vi "inputToGetList.vi"(8 "error in (no error)":errorcluster, 9 "NumOfDevices":i32, 10 "DeviceConnected":bool, 11 "SEDSpectrometer in":refnum<class "SEDSpectrometer.lvclass">) -> (0 "error out":errorcluster, 1 "ListInput":u8[](array[numeric]), 2 "ListSizeInput":i32, 3 "SEDSpectrometer out":refnum<class "SEDSpectrometer.lvclass">)   [LabVIEW 2016, in "SEDSpectrometer.lvclass"]
uses:
  SEDSpectrometer.lvclass
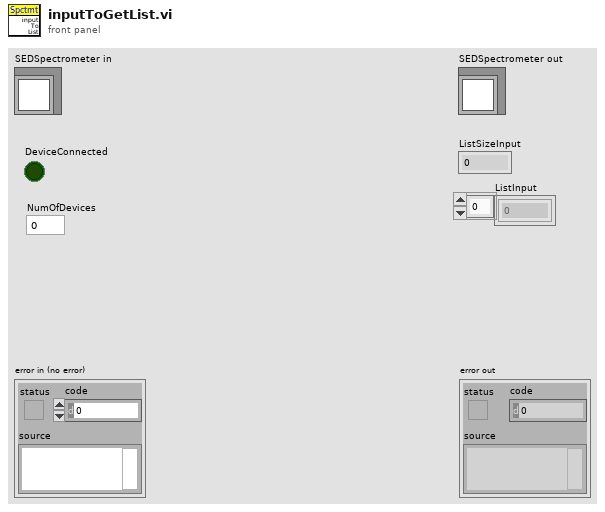
[diagram p1: front panel]
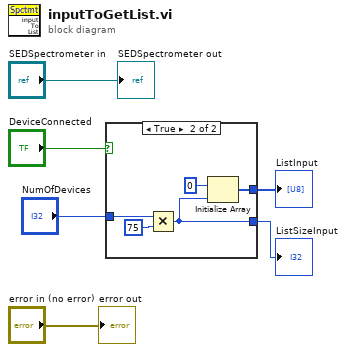
[diagram p0: block diagram]
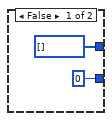
[diagram p2: hidden frame]
diagram:
  n1 = case shown="True" "DeviceConnected" {
    tunnel: "NumOfDevices" -> [_ w13]
    tunnel: [u8[] [] w10] -> w2
    tunnel: [0 w9] -> w1
    frame False {
    }
    frame True {
      n2 = Multiply(x=w13, y=75) -> (x*y=w9:i32)
      n3 = Initialize Array(u8 0, w9) -> (w10:u8[])
    }
  }
  "ListInput" <- w2
  "ListSizeInput" <- w1
  "error out" <- "error in (no error)"
  "SEDSpectrometer out" <- "SEDSpectrometer in"
